vi "Save-HFWM-Data.vi"(6 "Primary Line unit":enum16{"fs", "ps", "um", "mm", "counts"}(ring), 7 "Sample Channel Units":u16(ring), 8 "Data:  HFWM":dbl[][](array[numeric]), 9 "Secondary Delay":dbl[](array[numeric]), 10 "Primary Delay":dbl[](array[numeric]), 11 "Temperature":dbl[](array[numeric])) -> ()   [LabVIEW 2009]
panel:
  in  "Secondary Line unit":enum16{"fs", "ps", "um", "mm", "counts"}(ring)
  in  "size(s) temp":i32
  in  "size(s) delay":i32
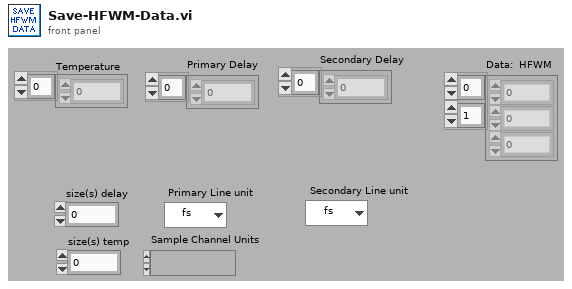
[diagram p1: front panel]
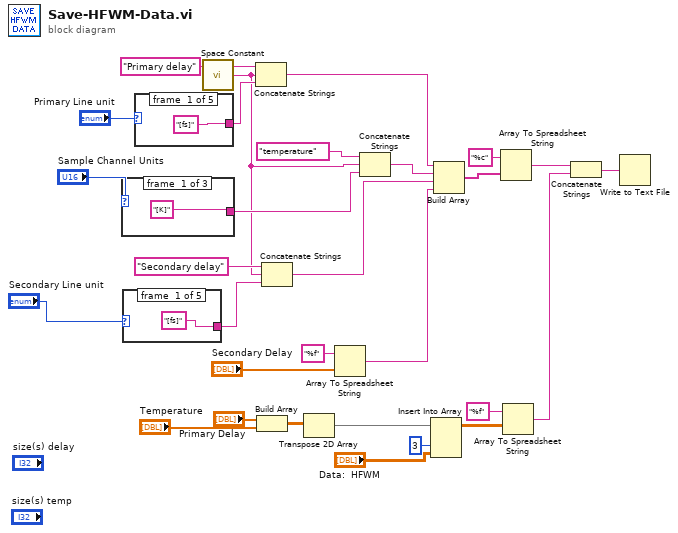
[diagram p0: block diagram]
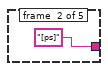
[diagram p2: hidden frame]
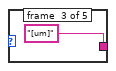
[diagram p3: hidden frame]
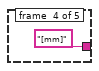
[diagram p4: hidden frame]
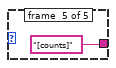
[diagram p5: hidden frame]
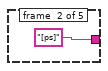
[diagram p6: hidden frame]
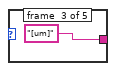
[diagram p7: hidden frame]
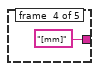
[diagram p8: hidden frame]
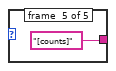
[diagram p9: hidden frame]
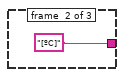
[diagram p10: hidden frame]
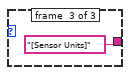
[diagram p11: hidden frame]
diagram:
  n1 = case shown="0, Default" "Sample Channel Units" {
    tunnel: ["[K]" "[ºC]" "[Sensor Units]"] -> w27
    frame #0 {
    }
    frame #1 {
    }
    frame #2 {
    }
  }
  n2 = case shown="\"counts\"" "Secondary Line unit" {
    tunnel: ["[fs]" "[ps]" "[um]" "[mm]" "[counts]"] -> w10
    frame #0 {
    }
    frame #1 {
    }
    frame #2 {
    }
    frame #3 {
    }
    frame #4 {
    }
  }
  n3 = case shown="\"counts\"" "Primary Line unit" {
    tunnel: ["[fs]" "[ps]" "[um]" "[mm]" "[counts]"] -> w21
    frame #0 {
    }
    frame #1 {
    }
    frame #2 {
    }
    frame #3 {
    }
    frame #4 {
    }
  }
  n4 = call <vilib>:"Space Constant.vi"() -> ("String"=w9:string)
  n5 = Concatenate Strings("Primary delay", w9, w21) -> (w7:string)
  n6 = Build Array("Primary Delay", "Temperature") -> (w18:dbl[][])
  n7 = Concatenate Strings("Secondary delay", w9, w10) -> (w5:string)
  n8 = Transpose 2D Array(2D array=w18) -> (transposed array=w16:dbl[][])
  n9 = Array To Spreadsheet String(array="Secondary Delay", 3:"%f" ("format string")) -> (spreadsheet string=w1:string)  [unwired: 1 in]
  n10 = Concatenate Strings("temperature", w9, w27) -> (w4:string)
  n11 = Insert Into Array(array=w16, index (col)=3 ("disabled index (col)"), new element="Data:  HFWM") -> (w14:dbl[][])  [unwired: 1 in]
  n12 = Build Array(w7, w4, w5, w1) -> (w24:string[])
  n13 = Array To Spreadsheet String(array=w24, 3:"%c" ("format string")) -> (spreadsheet string=w12:string)  [unwired: 1 in]
  n14 = Array To Spreadsheet String(array=w14, 3:"%f") -> (spreadsheet string=w17:string)  [unwired: 1 in]
  n15 = Concatenate Strings(w12, w17) -> (w6:string)
  n16 = Write to Text File(text=w6) -> ()  [unwired: 3 in, 3 out]
